vi "Update Waterfall.vi"(8 "error in":errorcluster, 11 "waterfall graph data out":T1={"z0"=0.0, "dz"=1.0, "plots"=[]}) -> (0 "error out":errorcluster)   [LabVIEW 2018, in "UDP Writer.lvlib"]
doc: "This subVI enqueues the named action in to the communications queue along with the input data."
uses:
  UDP Writer.lvlib
  Private Controls/Module Data.ctl
  Private Controls/Module Action.ctl
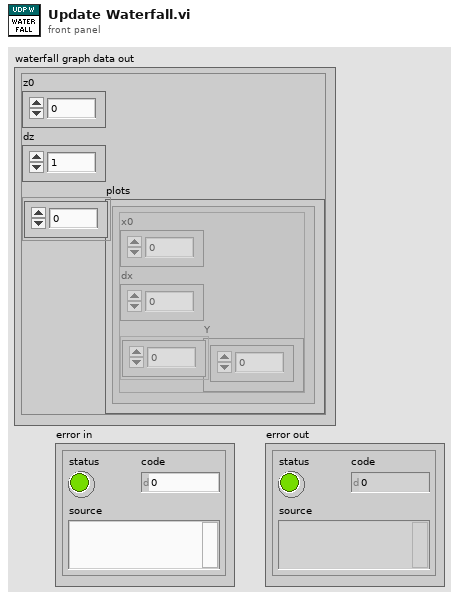
[diagram p1: front panel]
types:
  T1 = cluster{"z0":dbl, "dz":dbl, "plots":cluster{"x0":dbl, "dx":dbl, "Y":dbl[]}[]}
  T2 = typedef "UDP Writer.lvlib/Module Data.ctl" = cluster{"Data":variant, "Action":T3}
  T3 = typedef "UDP Writer.lvlib/Module Action.ctl" = enum16{"Init", "Update ARINC", "Update Waterfall", "Update RPMs", "Update Temps", "Update Modbus", "Update AI", "Update Vibs", "Write", "Error"}
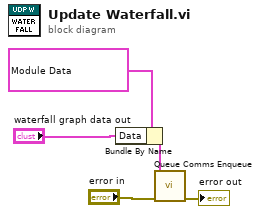
[diagram p0: block diagram]
diagram:
  n1 = Bundle By Name(cluster=T2 {"Data"=variant, "Action"=enum."Update Waterfall"} ("element"), "Data"="waterfall graph data out") -> (w2:T2)
  n2 = call "Queue Comms Enqueue.vi"("error in (no error)"="error in", "element"=w2) -> ("error out"=→"error out":errorcluster)  [unwired: 9 in]
